vi "Default Instrument Setup.vi"(8 "error in (no error)":errorcluster, 11 "VISA resource name":refnum<visa-resource-name>) -> (0 "error out":errorcluster, 3 "VISA resource name out":refnum<visa-resource-name>)   [LabVIEW 2015, in "BK Precision 983X Series.lvlib"]
doc: "This Utility VI sends a default command string to the instrument whenever a new VISA session is opened, or the instrument is reset. Use this VI as a subVI for the Initialize and Reset VIs. Altering this VI could cause these two VIs to operate incorrectly."
uses:
  <instrlib>/BK Precision 983X Series/BK Precision 983X Series.lvlib
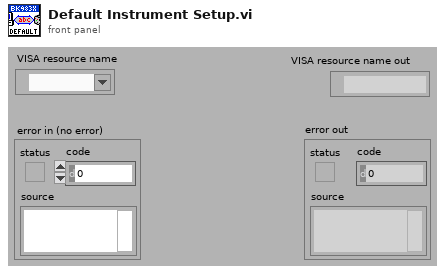
[diagram p1: front panel]
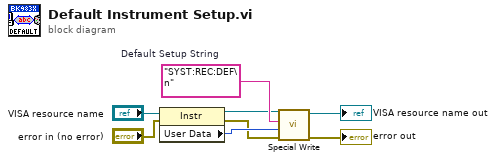
[diagram p0: block diagram]
diagram:
  w6 = "SYST:REC:DEF\n"  # Default Setup String
  n1 = property class="Instr"(reference="VISA resource name", error in="error in (no error)") -> (reference out=w1:refnum<visa-resource-name>, error out=w2:errorcluster, "User Data"=w3:u32)
  n2 = call <instrlib>:"Special Write.vi"("error in (no error)"=w2, "Delay (0 ms)"=w3, "Input String"=w6, "VISA resource name"=w1) -> ("error out"=→"error out":errorcluster, "VISA resource name out"=→"VISA resource name out":refnum<visa-resource-name>)  [unwired: 6 in]
